vi "Channel Measurement Trace Auto Scale.vi"(8 "error in (no error)":errorcluster {"code" format="%.0x"}, 9 "RepCapIdentifier":string, 11 "instrument handle":refnum<k15>) -> (0 "error out":errorcluster {"code" format="%.0x"}, 3 "instrument handle out":refnum<k15>)   [LabVIEW 2014, in "Agilent NA.lvlib"]
doc: "Performs autoscale on the selected trace"
uses:
  Agilent NA.lvlib
  AgNA.dll
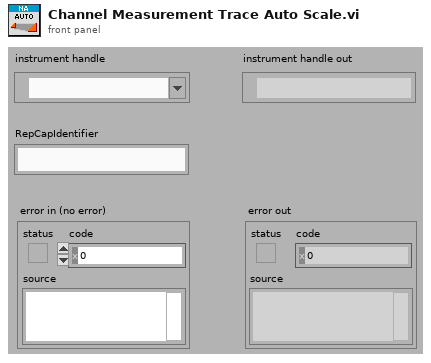
[diagram p1: front panel]
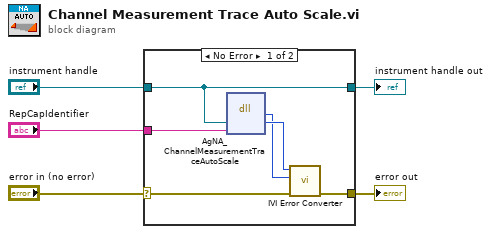
[diagram p0: block diagram]
diagram:
  n1 = case shown="No Error" "error in (no error)" {
    selector: "error in (no error)" -> [w9 w13]
    tunnel: [w8 w13] -> w5
    tunnel: "RepCapIdentifier" -> [w7 _]
    tunnel: [w6 w12] -> w2
    tunnel: "instrument handle" -> [w6 w12]
    frame No Error {
      n2 = dll-call lib="AgNA**.dll" fn="AgNA_ChannelMeasurementTraceAutoScale"("Vi"=w6, "RepCapIdentifier"=w7) -> (w10:i32, "Vi"=w11:u32)  [unwired: 4 in, 2 out]
      n3 = call "IVI Error Converter.vi"("error in (no error)"=w9, "IVI error code (0)"=w10, "instrument handle"=w11) -> ("error out"=w8:errorcluster)  [unwired: 7 in, 1 out]
    }
    frame Error {
    }
  }
  "error out" <- w5
  "instrument handle out" <- w2
